vi "Basic Manager Example.vi"() -> ()   [LabVIEW 2012, in "Phidget Manager.lvlib"]
uses:
  <instrlib>/Phidgets/Phidget Manager/Phidget Manager.lvlib
  <instrlib>/Phidgets/Phidget Common/Phidget Common.lvlib
panel:
  in  "Scan Time (ms)":u32=500
  out "DeviceInfo List":T1(array[cluster])
  out "Channel Class Names":string[](array[string])
  out "Channel Names":string[](array[string])
  out "Device Names":string[](array[string])
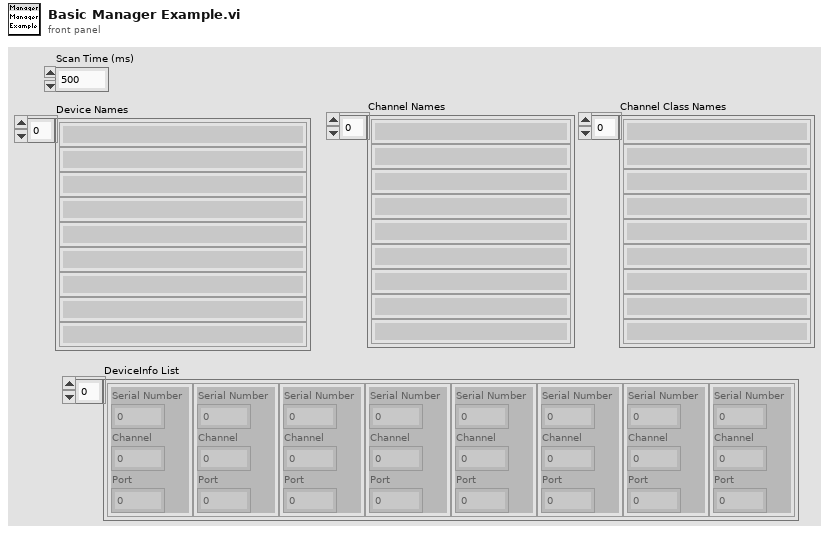
[diagram p1: front panel]
types:
  T1 = cluster{"Serial Number":i32, "Channel":i32, "Port":i32}[]
  T2 = cluster{"Serial Number":i32, "Channel":i32, "Port":i32}
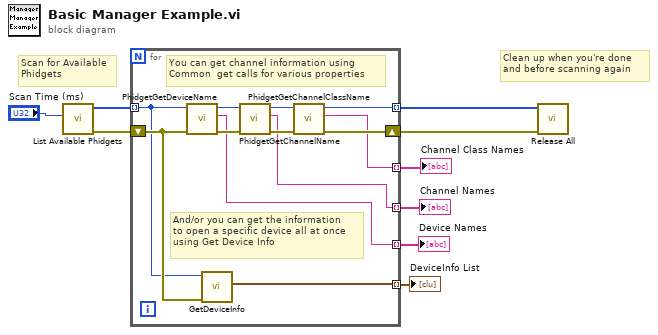
[diagram p0: block diagram]
diagram:
  # "Clean up when you're done\nand before scanning again"
  # "Scan for Available\nPhidgets"
  n1 = call <instrlib>:"List Available Phidgets.vi"("Timeout"="Scan Time (ms)") -> ("error out"=w5:errorcluster, "Available Handles"=w9:u64[])  [unwired: 9 in]
  n2 = for {
    tunnel: w9 -> [w13] mode=indexing
    tunnel: [w12] -> w8 mode=indexing
    tunnel: [w11] -> w7 mode=indexing
    tunnel: [w16] -> w6 mode=indexing
    shift-right: [w17] -> w4
    shift-left: w5 -> [w14]
    tunnel: [w15] -> w3 mode=indexing
    tunnel: [w10] -> w2 mode=indexing
    # "And/or you can get the information\nto open a specific device all at once\nusing Get Device Info"
    # "You can get channel information using\nCommon  get calls for various properties"
    n3 = call <instrlib>:"PhidgetGetDeviceName.vi"("error in"=w14, "Device In"=w13) -> ("error out"=w19:errorcluster, "DeviceName"=w12:string, "Device Out"=w21:u64)  [unwired: 7 in]
    n4 = call <instrlib>:"GetDeviceInfo.vi"("error in (no error)"=w14, "Device In"=w13) -> ("Device Info"=w10:T2)  [unwired: 4 in, 5 out]
    n5 = call <instrlib>:"PhidgetGetChannelName.vi"("error in"=w19, "Device In"=w21) -> ("error out"=w18:errorcluster, "ChannelName"=w11:string, "Device Out"=w20:u64)  [unwired: 7 in]
    n6 = call <instrlib>:"PhidgetGetChannelClassName.vi"("error in"=w18, "Device In"=w20) -> ("error out"=w17:errorcluster, "ChannelClassName"=w16:string, "Device Out"=w15:u64)  [unwired: 7 in]
  }
  "Device Names" <- w8
  "Channel Names" <- w7
  "Channel Class Names" <- w6
  "DeviceInfo List" <- w2
  n7 = call <instrlib>:"Release All.vi"("error in (no error)"=w4, "Available Handles"=w3) -> ()  [unwired: 9 in, 1 out]
